vi "Get Plot.vi"(9 "Stop":string, 10 "Start":string, 11 "Input String":string) -> (3 "Out String":string)   [LabVIEW 2024]
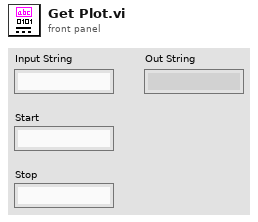
[diagram p1: front panel]
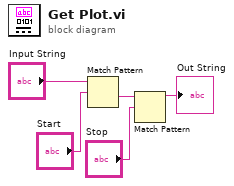
[diagram p0: block diagram]
diagram:
  n1 = Match Pattern(string="Input String", regular expression="Start") -> (after substring=w3:string)  [unwired: 1 in, 3 out]
  n2 = Match Pattern(string=w3, regular expression="Stop") -> (before substring=→"Out String":string)  [unwired: 1 in, 3 out]
